vi "ReadPort.vi"(8 "error in (no error)":errorcluster, 10 "PortRead":dbl, 11 "NXP in":refnum<class "NXP.lvclass">) -> (0 "error out":errorcluster, 3 "NXP out":refnum<class "NXP.lvclass">)   [LabVIEW 2020, in "NXP.lvclass"]
uses:
  NXP.lvclass
  Abstract/Serial Device/Serial Device.lvclass
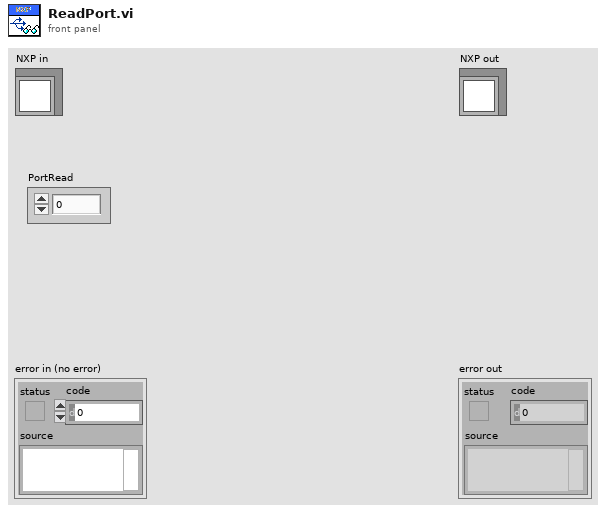
[diagram p1: front panel]
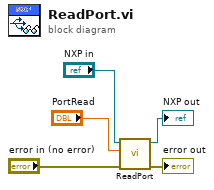
[diagram p0: block diagram]
diagram:
  n1 = call-parent "ReadPort.vi"("error in (no error)"="error in (no error)", "PortRead"="PortRead", "Serial Device in"="NXP in") -> ("error out"=→"error out":errorcluster, "Serial Device out"=→"NXP out":refnum<class "NXP.lvclass">)  [unwired: 7 in]
